vi "ReplaceZtoS.vi"(1 "String":string) -> (0 "result string":string)   [LabVIEW 2018]
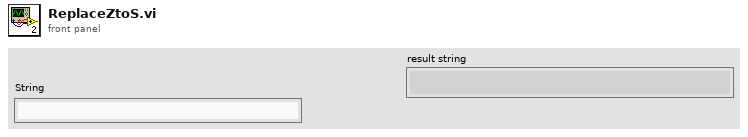
[diagram p1: front panel]
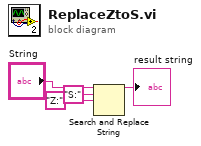
[diagram p0: block diagram]
diagram:
  n1 = Search and Replace String(input string="String", search string="S:", replace string="Z:" ("replace string (\"\")")) -> (result string=→"result string":string)  [unwired: 5 in, 3 out]
